vi "CombineGraphs.vi"() -> ()   [LabVIEW 2024]
uses:
  <userlib>/_OpenG.lib/array/array.llb/Conditional Auto-Indexing Tunnel (DBL)__ogtk.vi
  <userlib>/_OpenG.lib/array/array.llb/openg_array.lvlib
panel:
  in  "Tab Control":enum32{"Log Scale", "High", "Med", "Low"}(tab)
  in  "Output vs current":cluster{dbl[], dbl[]}[](graph)
  out "High Gain":cluster{dbl[], dbl[]}(graph)
  out "Med Gain":cluster{dbl[], dbl[]}(graph)
  out "Low Gain":cluster{dbl[], dbl[]}(graph)
  out "Array 2":dbl[][](array[numeric])
  out "Array":dbl[][](array[numeric])
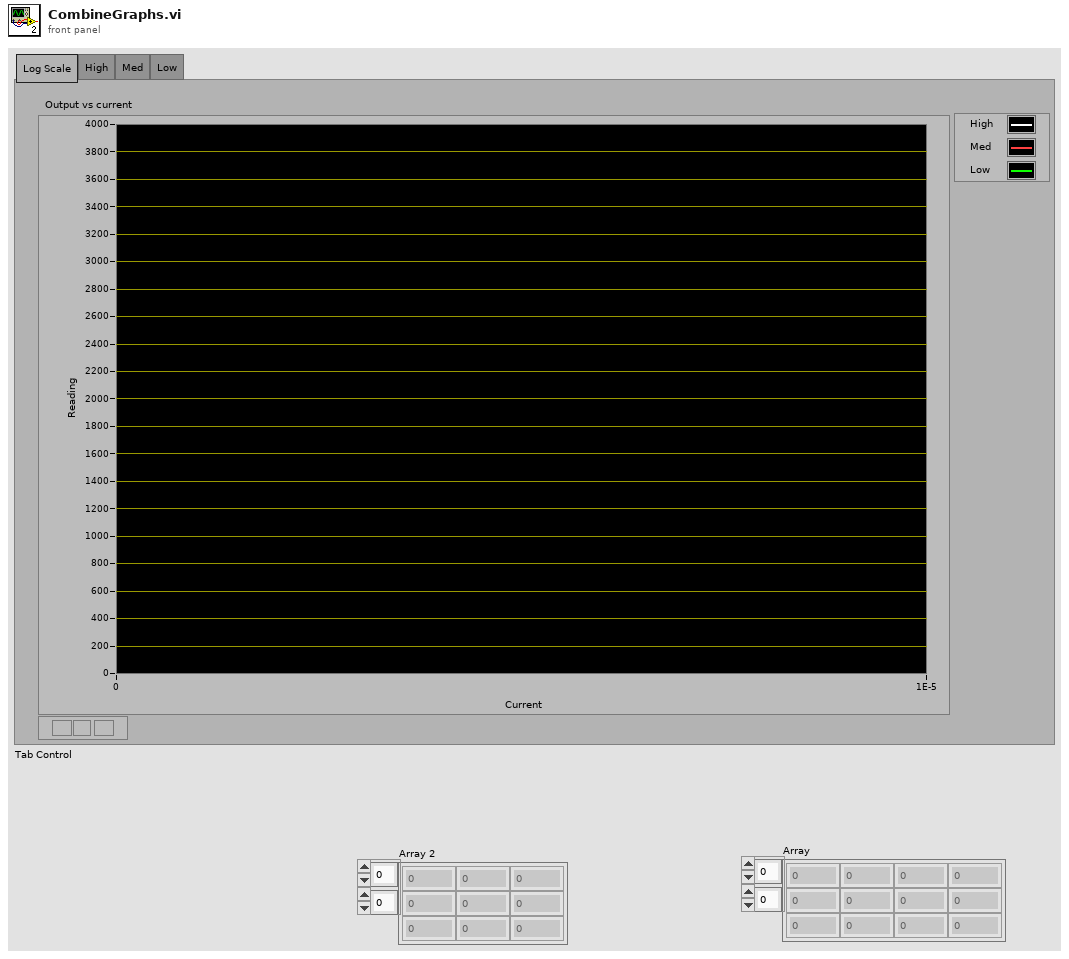
[diagram p1: front panel]
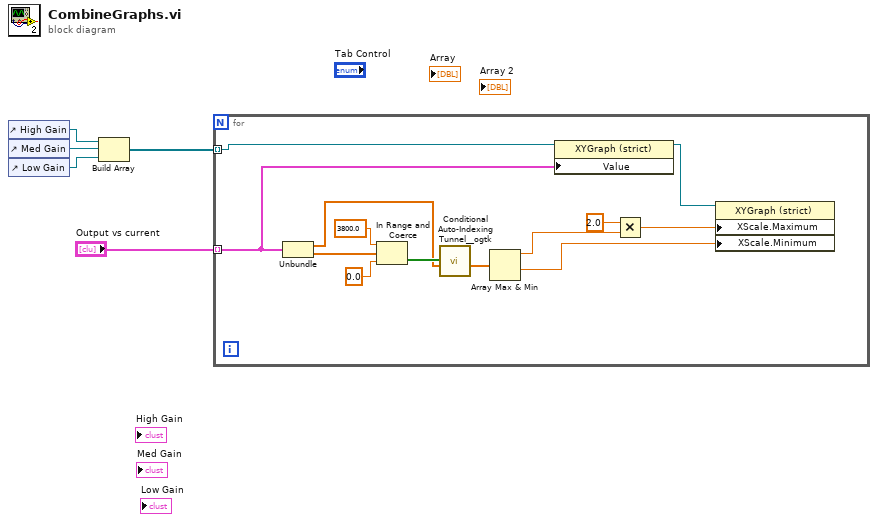
[diagram p0: block diagram]
diagram:
  n1 = control-ref of="High Gain"() -> (w3:refnum<vi>)
  n2 = control-ref of="Med Gain"() -> (w4:refnum<vi>)
  n3 = control-ref of="Low Gain"() -> (w2:refnum<vi>)
  n4 = Build Array(w3, w4, w2) -> (w1:refnum<vi>[])
  n5 = for {
    tunnel: "Output vs current" -> [w12] mode=indexing
    tunnel: w1 -> [w10] mode=indexing
    n6 = Unbundle(w12) -> (w14:dbl[], w18:dbl[])
    n7 = In Range and Coerce(upper limit=3800.0, x=w18, lower limit=0.0) -> (In Range?=w15:bool[])  [unwired: 1 out]
    n8 = call-poly <userlib>:"Conditional Auto-Indexing Tunnel__ogtk.vi"("Array in"=w14, "Elements to keep"=w15) -> ("Filtered Array out"=w13:dbl[])  [unwired: 5 in]
    n9 = Array Max & Min(array=w13) -> (max value=w7:dbl, min value=w9:dbl)  [unwired: 2 out]
    n10 = property on="Property Node" class="XYGraph (strict)"(reference=w10, "Value"=w12) -> (reference out=w11:refnum<vi>)  [unwired: 1 in, 1 out]
    n11 = Multiply(x=2.0, y=w7) -> (x*y=w8:dbl)
    n12 = property on="Property Node" class="XYGraph (strict)"(reference=w11, "XScale.Maximum"=w8, "XScale.Minimum"=w9) -> ()  [unwired: 1 in, 2 out]
  }
